vi "Make Waveform Time Array.vi"(6 "Actual size":i32, 8 "error in (no error)":errorcluster, 11 "waveform in":waveform(sgl)) -> (0 "error out":errorcluster, 2 "X array":dbl[](array[numeric]) format="%#_15g")   [LabVIEW 2015]
doc: "Creates an array of waveform time stamps. Each element in the array is the time stamp for each data value in the waveform. Wire data to the <B>waveform in</B> input to determine the polymorphic instance to use or manually select the instance."
uses:
  <vilib>/Waveform/WDTOps.llb/WDT Number of Waveform Samples SGL.vi
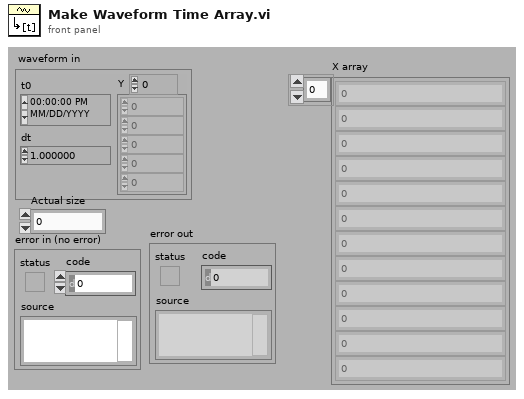
[diagram p1: front panel]
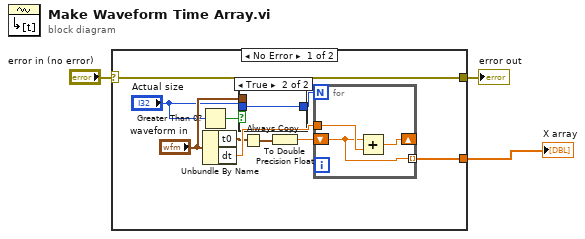
[diagram p0: block diagram]
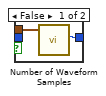
[diagram p2: hidden frame]
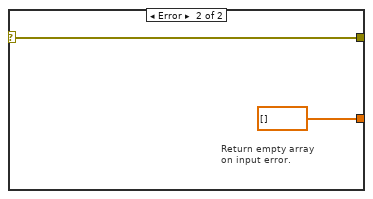
[diagram p3: hidden frame]
diagram:
  n1 = case shown="No Error" "error in (no error)" {
    selector: "error in (no error)" -> [w9 w21]
    tunnel: [w10 sgl[] [] ("X array")] -> w3
    tunnel: [w9 w21] -> w2
    frame No Error {
      n2 = Greater Than 0?(x="Actual size") -> (x > 0?=w5:bool)
      n3 = Unbundle By Name("waveform in") -> ("t0"=w8:timestamp, "dt"=w11:dbl)
      n4 = Always Copy(1:w8) -> (0:w7:timestamp)
      n5 = case shown="True" w5 {
        tunnel: [w15 w16] -> w13
        tunnel: "waveform in" -> [w14 _]
        tunnel: "Actual size" -> [_ w16]
        frame False {
          n6 = call-poly <vilib>:"Number of Waveform Samples.vi"("waveform in"=w14) -> ("number of samples"=w15:i32)  [unwired: 1 in, 9 out]
        }
        frame True {
        }
      }
      n7 = To Double Precision Float(number=w7) -> (double precision float=w6:dbl)
      n8 = for {
        N: w13 -> [_]
        shift-right: [w18] -> _
        shift-left: w6 -> [w17]
        tunnel: w11 -> [w19]
        tunnel: [w17] -> w10 mode=indexing
        n9 = Add(x=w17, y=w19) -> (x+y=w18:dbl)
      }
    }
    frame Error {
      # "Return empty array\non input error."
    }
  }
  "error out" <- w2
  "X array" <- w3
